vi "REL_move.vi"() -> ()   [LabVIEW 2019]
doc: "This example demonstrate how to run drive with Absolute."
uses:
  <vilib>/addons/eal4LabVIEW/ApiLib/Connection control/ealApiConnect_string.vi
  <vilib>/addons/eal4LabVIEW/eal4LabVIEW.lvlib
panel:
  in  "Parameter set 3 for MoveAbsolute":T1={"Position"=4000.0, "Velocity"=100.0, "Acceleration"=0.0, "Deceleration"=0.0, "Jerk"=0.0}
  in  "Parameter set 2 for relmove":T1={"Position"=8000.0, "Velocity"=500.0, "Acceleration"=100.0, "Deceleration"=10.0, "Jerk"=0.0}
  in  "Parameter set 1 for MoveAbsolute":T1={"Position"=2000.0, "Velocity"=200.0, "Acceleration"=1.0, "Deceleration"=10.0, "Jerk"=0.0}
  in  "IP address":string="172.17.24.139"
  # "THIAGARAJAR COLLEGE OF ENGINEERING\n      Department of Mechatronics Engineering"
  # "Waits for 10 seconds\nbefore applying next set."
  # "Waits for 10 seconds\nbefore applying next set."
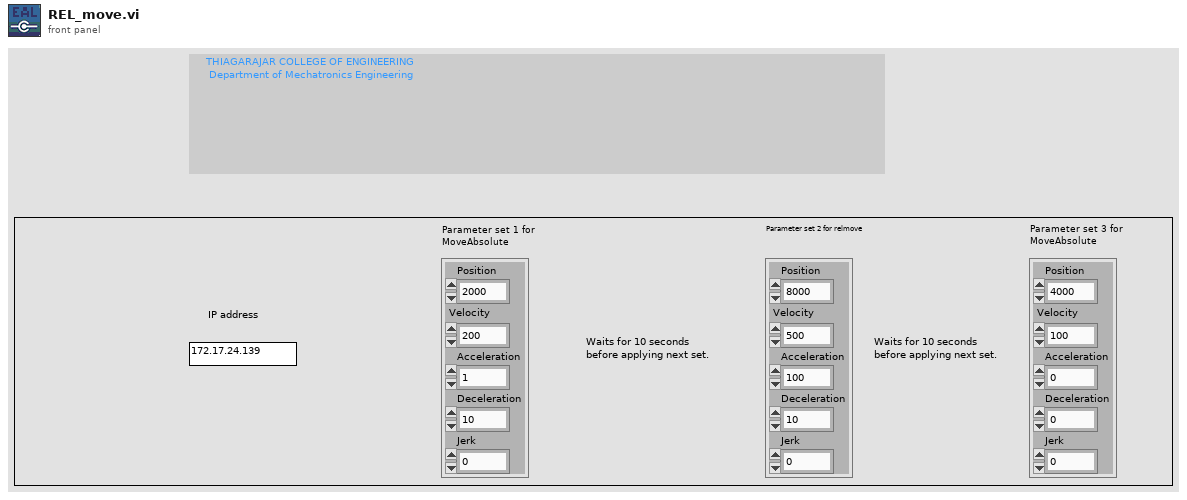
[diagram p1: front panel]
types:
  T1 = cluster{"Position":dbl, "Velocity":dbl, "Acceleration":dbl, "Deceleration":dbl, "Jerk":dbl}
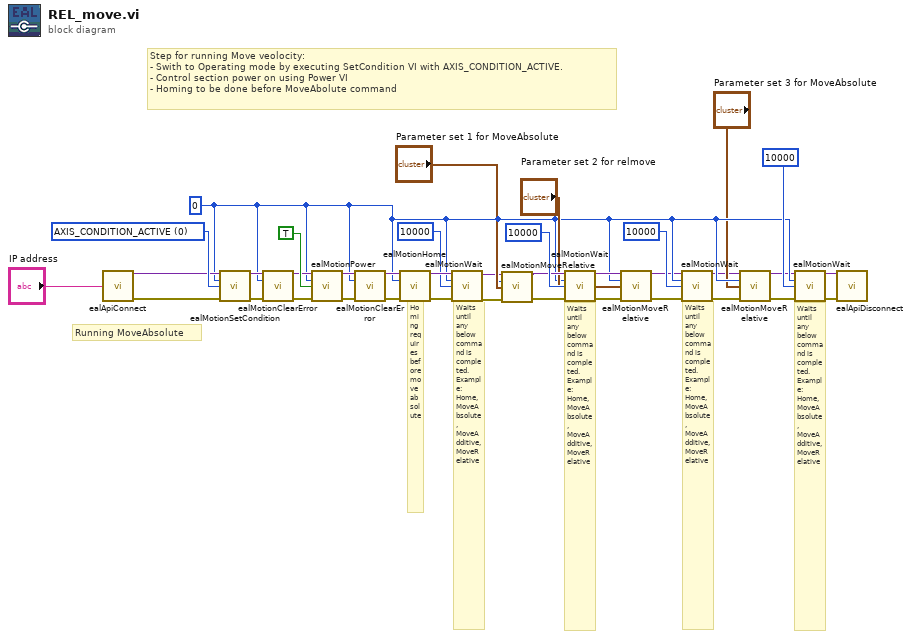
[diagram p0: block diagram]
diagram:
  w8 = 0 ("slave index")
  w35 = 0 items=["AXIS_CONDITION_ACTIVE"=0, "AXIS_CONDITION_PARKING"=1, "AXIS_CONDITION_DEACTIVATED"=2, "AXIS_CONDITION_ACTIVE_DECOUPLED"=4, "AXIS_CONDITION_PARKING_DECOUPLED"=5, "AXIS_CONDITION_DEACTIVATED_DECOUPLED"=6, "AXIS_CONDITION_ACTIVE_PARAMETERIZATION"=8, "AXIS_CONDITION_PARKING_PARAMETERIZATION"=9, "AXIS_CONDITION_DEACTIVATED_PARAMETERIZATION"=10, "AXIS_CONDITION_ACTIVE_DECOUPLED_PARAMETERIZATION"=12, "AXIS_CONDITION_PARKING_DECOUPLED_PARAMETERIZATION"=13, "AXIS_CONDITION_DEACTIVATED_DECOUPLED_PARAMETERIZATION"=14] ("condition")
  # "Waits until any below command is completed.\nExample: Home, MoveAbsolute, MoveAdditive, MoveRelative"
  # "Waits until any below command is completed.\nExample: Home, MoveAbsolute, MoveAdditive, MoveRelative"
  # "Waits until any below command is completed.\nExample: Home, MoveAbsolute, MoveAdditive, MoveRelative"
  # "Waits until any below command is completed.\nExample: Home, MoveAbsolute, MoveAdditive, MoveRelative"
  # "Homing requires before move absolute"
  # "Running MoveAbsolute"
  # "Step for running Move veolocity:\n- Swith to Operating mode by executing SetCondition VI with AXIS_CONDITION_ACTIVE.\n- Control section power on using Power VI\n- Homing to be done before MoveAbolute command"
  n1 = call-poly <vilib>:"ealApiConnect.vi"("ip address"="IP address") -> ("connection out"=w28:variant, "error out"=w27:errorcluster)  [unwired: 13 in]
  n2 = call <vilib>:"ealMotionSetCondition.vi"("connection in"=w28, "slave index"=w8, "condition"=w35, "error in (no error)"=w27) -> ("connection out"=w34:variant, "error out"=w33:errorcluster)  [unwired: 10 in]
  n3 = call <vilib>:"ealMotionClearError.vi"("connection in"=w34, "slave index"=w8, "error in (no error)"=w33) -> ("connection out"=w32:variant, "error out"=w31:errorcluster)  [unwired: 11 in]
  n4 = call <vilib>:"ealMotionPower.vi"("connection in"=w32, "slave index"=w8, "value"=TRUE, "error in (no error)"=w31) -> ("connection out"=w29:variant, "error out"=w30:errorcluster)  [unwired: 10 in]
  n5 = call <vilib>:"ealMotionClearError.vi"("connection in"=w29, "slave index"=w8, "error in (no error)"=w30) -> ("connection out"=w26:variant, "error out"=w25:errorcluster)  [unwired: 11 in]
  n6 = call <vilib>:"ealMotionHome.vi"("connection in"=w26, "slave index"=w8, "error in (no error)"=w25) -> ("connection out"=w24:variant, "error out"=w23:errorcluster)  [unwired: 11 in]
  n7 = call <vilib>:"ealMotionWait.vi"("connection in"=w24, "slave index"=w8, "timeout"=10000, "error in (no error)"=w23) -> ("connection out"=w12:variant, "error out"=w13:errorcluster)  [unwired: 10 in]
  n8 = call <vilib>:"ealMotionMoveRelative.vi"("connection in"=w12, "slave index"=w8, "parameters set"="Parameter set 1 for MoveAbsolute", "error in (no error)"=w13) -> ("connection out"=w15:variant, "error out"=w16:errorcluster)  [unwired: 10 in]
  n9 = call <vilib>:"ealMotionWait.vi"("connection in"=w15, "slave index"=w8, "timeout"=10000, "error in (no error)"=w16) -> ("connection out"=w10:variant, "error out"=w9:errorcluster)  [unwired: 10 in]
  n10 = call <vilib>:"ealMotionMoveRelative.vi"("connection in"=w10, "slave index"=w8, "parameters set"="Parameter set 2 for relmove", "error in (no error)"=w9) -> ("connection out"=w1:variant, "error out"=w2:errorcluster)  [unwired: 10 in]
  n11 = call <vilib>:"ealMotionWait.vi"("connection in"=w1, "slave index"=w8, "timeout"=10000, "error in (no error)"=w2) -> ("connection out"=w6:variant, "error out"=w5:errorcluster)  [unwired: 10 in]
  n12 = call <vilib>:"ealMotionMoveRelative.vi"("connection in"=w6, "slave index"=w8, "parameters set"="Parameter set 3 for MoveAbsolute", "error in (no error)"=w5) -> ("connection out"=w4:variant, "error out"=w3:errorcluster)  [unwired: 10 in]
  n13 = call <vilib>:"ealMotionWait.vi"("connection in"=w4, "slave index"=w8, "timeout"=10000, "error in (no error)"=w3) -> ("connection out"=w22:variant, "error out"=w21:errorcluster)  [unwired: 10 in]
  n14 = call <vilib>:"ealApiDisconnect.vi"("connection in"=w22, "error in (no error)"=w21) -> ()  [unwired: 13 in, 1 out]
